vi "Set Measurment Parameters(SubVI).vi"(0 "Handle In":T1 {"Handle" format="0x%08x"; "Conn" format="0x%08x"}, 1 "Parameters":T2={"model"=1, "auto/output"=FALSE, "output/amplitude"=0.1, "current/range"=0.001, "voltage/range"=1.0, "auto/inputrange"=FALSE, "mode"=1} {"mode" items=["4-terminal", "2-terminal"]; "model" items=["Rp || Cp", "Rs + Cs", "Rs + Ls", "G B", "D Cs", "Q Cs", "D Ls", "Q Ls", "Rp || Lp", "D Cp"]}, 2 "Pause time":u32=500, 3 "Error In":errorcluster, 4 "Enable compensation":bool) -> (5 "Handle Out":T1 {"Handle" format="0x%08x"; "Conn" format="0x%08x"}, 6 "Error Out":errorcluster)   [LabVIEW 2019]
doc: "This VI is used to set equivalent circuit, test signal level and voltage and current ranges."
uses:
  <instrlib>/Zurich Instruments LabOne/Public/ziTypeHandle.ctl
  <instrlib>/Zurich Instruments LabOne/Public/Configure/ziSetValueDoubleArray.vi
  <instrlib>/Zurich Instruments LabOne/Public/Configure/ziSetValueDouble.vi
  <instrlib>/Zurich Instruments LabOne/Zurich Instruments LabOne.lvlib
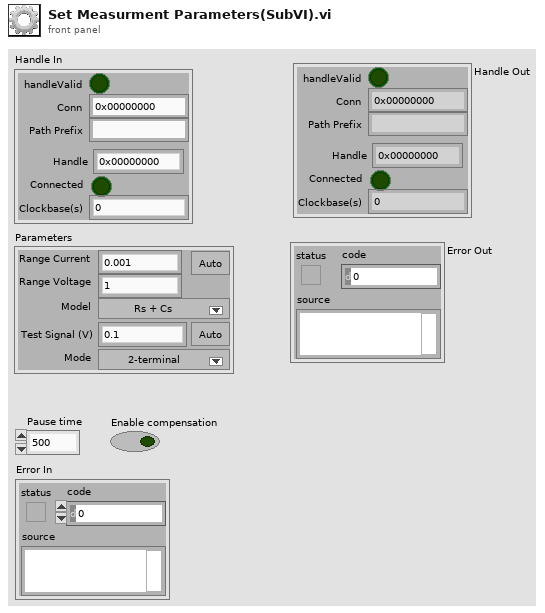
[diagram p1: front panel]
types:
  T1 = typedef "Zurich Instruments LabOne.lvlib/ziTypeHandle.ctl" = cluster{"handleValid":bool, "Conn":u64, "Path Prefix":string, "Handle":u64, "Connected":bool, "Clockbase(s)":dbl}
  T2 = cluster{"model":u16, "auto/output":bool, "output/amplitude":dbl, "current/range":dbl, "voltage/range":dbl, "auto/inputrange":bool, "mode":u16}
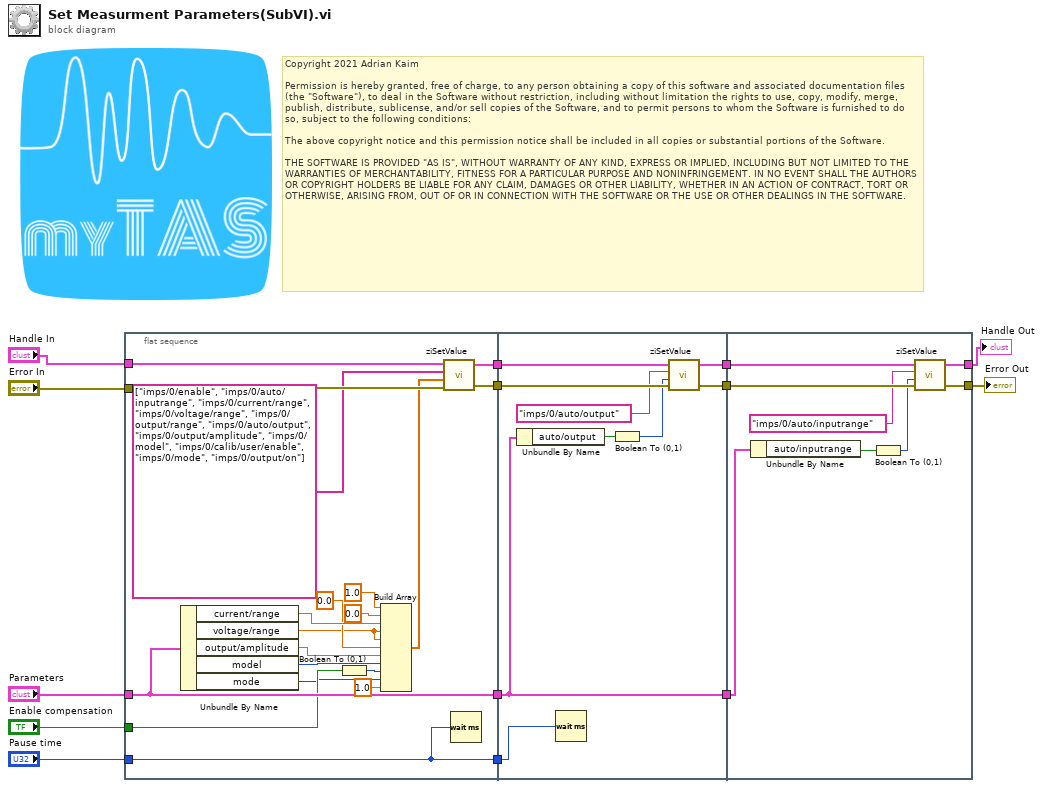
[diagram p0: block diagram]
diagram:
  # "Copyright 2021 Adrian Kaim\n\nPermission is hereby granted, free of charge, to any person obtaining a copy of this software and associated documentation files (the \"Software\"), to deal in the Software without restriction, including without limitation the rights to use, copy, modify, merge, publish, distribute, sublicense, and/or sell copies of the Software, and to permit persons to whom the Software is furnished to do so, subject to the following conditions:\n\nThe above copyright notice and this permission notice shall be included in all copies or substantial portions of the Software.\n\nTHE SOFTWARE IS PROVIDED \"AS IS\", WITHOUT WARRANTY OF ANY KIND, EXPRESS OR IMPLIED, INCLUDING BUT NOT LIMITED TO THE WARRANTIES OF MERCHANTABILITY, FITNESS FOR A PARTICULAR PURPOSE AND NONINFRINGEMENT. IN NO EVENT SHALL THE AUTHORS OR COPYRIGHT HOLDERS BE LIABLE FOR ANY CLAIM, DAMAGES OR OTHER LIABILITY, WHETHER IN AN ACTION OF CONTRACT, TORT OR OTHERWISE, ARISING FROM, OUT OF OR IN CONNECTION WITH THE SOFTWARE OR THE USE OR OTHER DEALINGS IN THE SOFTWARE."
  n1 = flat-sequence {
    tunnel: "Error In" -> [w33]
    tunnel: "Handle In" -> [w32]
    tunnel: [w31] -> w12
    tunnel: [w30] -> w11
    tunnel: "Parameters" -> [w22]
    tunnel: [w22] -> w4
    tunnel: [w20] -> w3
    tunnel: "Pause time" -> [w20]
    tunnel: "Enable compensation" -> [w18]
    tunnel: w12 -> [w42]
    tunnel: w11 -> [w41]
    tunnel: [w40] -> w7
    tunnel: [w39] -> w6
    tunnel: [w38] -> w5
    tunnel: w4 -> [w38]
    tunnel: w3 -> [w34]
    tunnel: [w48] -> w9
    tunnel: [w47] -> w10
    tunnel: w7 -> [w50]
    tunnel: w6 -> [w49]
    tunnel: w5 -> [w46]
    frame #0 {
      n2 = Unbundle By Name(w22) -> ("current/range"=w27:dbl, "voltage/range"=w16:dbl, "output/amplitude"=w28:dbl, "model"=w21:u16, "mode"=w17:u16)
      n3 = Boolean To (0,1)(Boolean=w18) -> (0, 1=w19:i16)
      n4 = Build Array(1.0 ("element"), 0.0 ("element"), w27, w16, w16, 0.0 ("element"), w28, w21, w19, w17, 1.0 ("element")) -> (w23:dbl[])
      n5 = call-poly <instrlib>:"ziSetValue.vi"("Error In"=w33, "Values"=w23, "Paths"=string[] ["imps/0/enable", "imps/0/auto/inputrange", "imps/0/current/range", "imps/0/voltage/range", "imps/0/output/range", "imps/0/auto/output", "imps/0/output/amplitude", "imps/0/model", "imps/0/calib/user/enable", "imps/0/mode", "imps/0/output/on"], "Handle In"=w32) -> ("Error Out"=w30:errorcluster, "Handle Out"=w31:T1)  [unwired: 1 in]
      n6 = Wait (ms)(milliseconds to wait=w20) -> ()  [unwired: 1 out]
    }
    frame #1 {
      n7 = Unbundle By Name(w38) -> ("auto/output"=w37:bool)
      n8 = Wait (ms)(milliseconds to wait=w34) -> ()  [unwired: 1 out]
      n9 = Boolean To (0,1)(Boolean=w37) -> (0, 1=w35:i16)
      n10 = call-poly <instrlib>:"ziSetValue.vi"("Error In"=w41, "Value"=w35, "Path"="imps/0/auto/output", "Handle In"=w42) -> ("Error Out"=w39:errorcluster, "Handle Out"=w40:T1)  [unwired: 1 in]
    }
    frame #2 {
      n11 = Unbundle By Name(w46) -> ("auto/inputrange"=w44:bool)
      n12 = Boolean To (0,1)(Boolean=w44) -> (0, 1=w43:i16)
      n13 = call-poly <instrlib>:"ziSetValue.vi"("Error In"=w49, "Value"=w43, "Path"="imps/0/auto/inputrange", "Handle In"=w50) -> ("Error Out"=w48:errorcluster, "Handle Out"=w47:T1)  [unwired: 1 in]
    }
  }
  "Handle Out" <- w10
  "Error Out" <- w9
